vi "Forward Lockin Result to Output.vi"(8 "error in (no error)":errorcluster, 10 "Waveforms [] in":waveform(dbl)[](array[waveform]), 11 "Generator in":refnum<class "Generator.lvclass">) -> (0 "error out":errorcluster, 2 "Waveforms [] out":waveform(dbl)[](array[waveform]), 3 "Generator out":refnum<class "Generator.lvclass">)   [LabVIEW 2019, in "Generator.lvclass"]
uses:
  Generator.lvclass
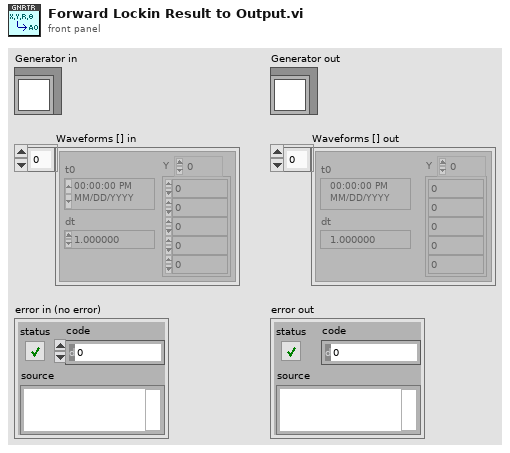
[diagram p1: front panel]
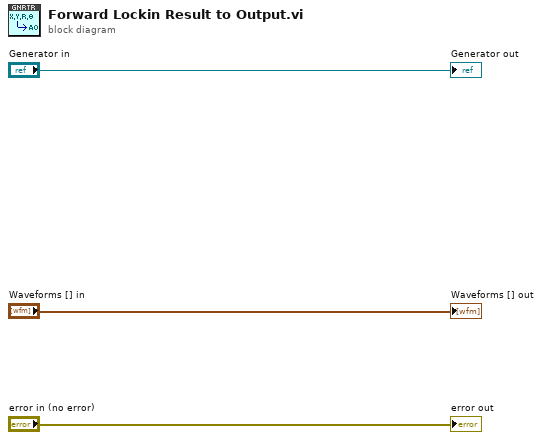
[diagram p0: block diagram]
diagram:
  "Waveforms [] out" <- "Waveforms [] in"
  "Generator out" <- "Generator in"
  "error out" <- "error in (no error)"
